vi "HV Kill Channels.vi"() -> ()   [LabVIEW 2018, in "HV QMH.lvlib"]
uses:
  HV QMH.lvlib
panel:
  out "Output":string
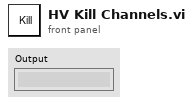
[diagram p1: front panel]
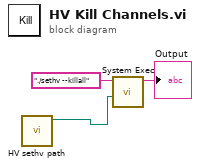
[diagram p0: block diagram]
diagram:
  n1 = call "HV sethv path.vi"() -> ("sethv filepath"=w1:path)  [unwired: 11 in]
  n2 = call <vilib>:"System Exec.vi"("working directory"=w1, "command line"="./sethv --killall") -> ("standard output"=→"Output":string)  [unwired: 6 in, 3 out]
